vi "interface.vi"() -> ()   [LabVIEW 2009]
uses:
  <vilib>/Instr/_visa.llb/VISA Configure Serial Port (Instr).vi
panel:
  out "Thermometer":dbl(slide) scale=0.0..100.0
  out "Waveform Chart":dbl(graph)
  in  "stop":bool
  in  "VISA resource name":refnum<visa-resource-name>
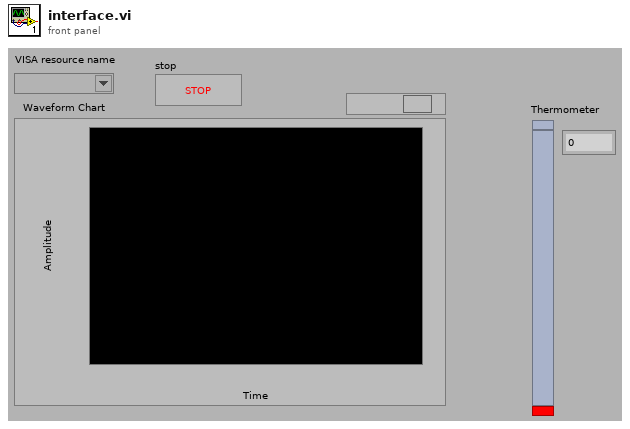
[diagram p1: front panel]
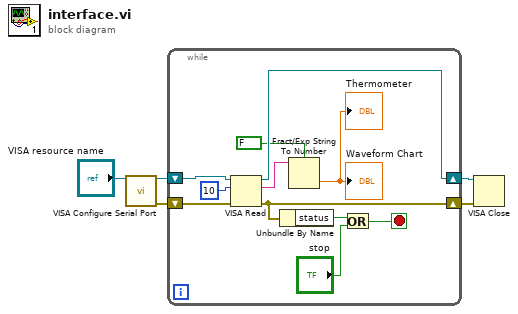
[diagram p0: block diagram]
diagram:
  n1 = call-poly "VISA Configure Serial Port"("VISA resource name"="VISA resource name") -> ("VISA resource name out"=w4:refnum<visa-resource-name>, "error out"=w3:errorcluster)  [unwired: 13 in]
  n2 = while {
    shift-right: [w11] -> w1
    shift-left: w3 -> [w15]
    shift-right: [w12] -> w2
    shift-left: w4 -> [w16]
    stop <- w8 stop-if-true
    n3 = VISA Read(VISA resource name=w16, byte count=u32 10, error in (no error)=w15) -> (VISA resource name out=w12:refnum<visa-resource-name>, read buffer=w13:string, error out=w11:errorcluster)  [unwired: 1 out]
    n4 = Unbundle By Name(w11) -> ("status"=w10:bool)
    n5 = Fract/Exp String To Number(use system decimal point (T)=FALSE, string=w13) -> (number=→"Waveform Chart" →"Thermometer":dbl)  [unwired: 2 in, 1 out]
    n6 = Or(x=w10, y="stop") -> (x .or. y?=w8:bool)
  }
  n7 = VISA Close(VISA resource name=w2, error in (no error)=w1) -> ()  [unwired: 1 out]
